vi "ATF-Pumb HW Splitter.vi"(10 "data":T1={"AO config"=[], "AI config"=[], "DI config"=[], "DO config"=[], "TC config"=[], "ACC config"=[], "SG config"=[], "Strain Gauge Settings"={"poisson ratio"=0.3, "nominal gage resistance"=120.0, "gage factor"=2.08}, "Bridge Settings"={"voltage excitation value"=3.3, "voltage excitation source"=10200, "initial bridge voltage"=0.0, "lead wire resistance"=1.7, "strain configuration"=10271}, "Sample Rate"={"AI Sample Rate"=[], "AO Sample Rate"=[], "DI Sample Rate"=[], "TC Sample Rate"=[], "DO Sample Rate"=[], "SG Sample Rate"=[], "ACC Sample Rate"=[]}} {"Bridge Settings"."strain configuration" items=["Full Bridge I"=10183, "Full Bridge II"=10184, "Full Bridge III"=10185, "Half Bridge I"=10188, "Half Bridge II"=10189, "Quarter Bridge I"=10271, "Quarter Bridge II"=10272]; "Bridge Settings"."voltage excitation source" items=["Internal"=10200, "External"=10167, "None"=10230]; "ACC config"."Terminal configuration" items=["default"=-1, "RSE"=10083, "NRSE"=10078, "Differential"=10106, "Pseudodifferential"=12529]; "ACC config"."Sensitivity units" items=["mVolts/g"=12509, "Volts/g"=12510]; "TC config"."type" items=["J"=10072, "K"=10073, "N"=10077, "R"=10082, "S"=10085, "T"=10086, "B"=10047, "E"=10055]; "TC config"."units" items=["Deg C", "Deg F", "Kelvins", "Deg R", "From Custom Scale"]}, 11 "Pumb Expression":string="cRIO") -> (1 "Pumb HW":T1={"AO config"=[], "AI config"=[], "DI config"=[], "DO config"=[], "TC config"=[], "ACC config"=[], "SG config"=[], "Strain Gauge Settings"={"poisson ratio"=0.3, "nominal gage resistance"=120.0, "gage factor"=2.08}, "Bridge Settings"={"voltage excitation value"=3.3, "voltage excitation source"=10200, "initial bridge voltage"=0.0, "lead wire resistance"=1.7, "strain configuration"=10271}, "Sample Rate"={"AI Sample Rate"=[], "AO Sample Rate"=[], "DI Sample Rate"=[], "TC Sample Rate"=[], "DO Sample Rate"=[], "SG Sample Rate"=[], "ACC Sample Rate"=[]}} {"Bridge Settings"."strain configuration" items=["Full Bridge I"=10183, "Full Bridge II"=10184, "Full Bridge III"=10185, "Half Bridge I"=10188, "Half Bridge II"=10189, "Quarter Bridge I"=10271, "Quarter Bridge II"=10272]; "Bridge Settings"."voltage excitation source" items=["Internal"=10200, "External"=10167, "None"=10230]; "ACC config"."Terminal configuration" items=["default"=-1, "RSE"=10083, "NRSE"=10078, "Differential"=10106, "Pseudodifferential"=12529]; "ACC config"."Sensitivity units" items=["mVolts/g"=12509, "Volts/g"=12510]; "TC config"."type" items=["J"=10072, "K"=10073, "N"=10077, "R"=10082, "S"=10085, "T"=10086, "B"=10047, "E"=10055]; "TC config"."units" items=["Deg C", "Deg F", "Kelvins", "Deg R", "From Custom Scale"]}, 3 "Storage HW":T1={"AO config"=[], "AI config"=[], "DI config"=[], "DO config"=[], "TC config"=[], "ACC config"=[], "SG config"=[], "Strain Gauge Settings"={"poisson ratio"=0.3, "nominal gage resistance"=120.0, "gage factor"=2.08}, "Bridge Settings"={"voltage excitation value"=3.3, "voltage excitation source"=10200, "initial bridge voltage"=0.0, "lead wire resistance"=1.7, "strain configuration"=10271}, "Sample Rate"={"AI Sample Rate"=[], "AO Sample Rate"=[], "DI Sample Rate"=[], "TC Sample Rate"=[], "DO Sample Rate"=[], "SG Sample Rate"=[], "ACC Sample Rate"=[]}} {"Bridge Settings"."strain configuration" items=["Full Bridge I"=10183, "Full Bridge II"=10184, "Full Bridge III"=10185, "Half Bridge I"=10188, "Half Bridge II"=10189, "Quarter Bridge I"=10271, "Quarter Bridge II"=10272]; "Bridge Settings"."voltage excitation source" items=["Internal"=10200, "External"=10167, "None"=10230]; "ACC config"."Terminal configuration" items=["default"=-1, "RSE"=10083, "NRSE"=10078, "Differential"=10106, "Pseudodifferential"=12529]; "ACC config"."Sensitivity units" items=["mVolts/g"=12509, "Volts/g"=12510]; "TC config"."type" items=["J"=10072, "K"=10073, "N"=10077, "R"=10082, "S"=10085, "T"=10086, "B"=10047, "E"=10055]; "TC config"."units" items=["Deg C", "Deg F", "Kelvins", "Deg R", "From Custom Scale"]})   [LabVIEW 2022 SP3]
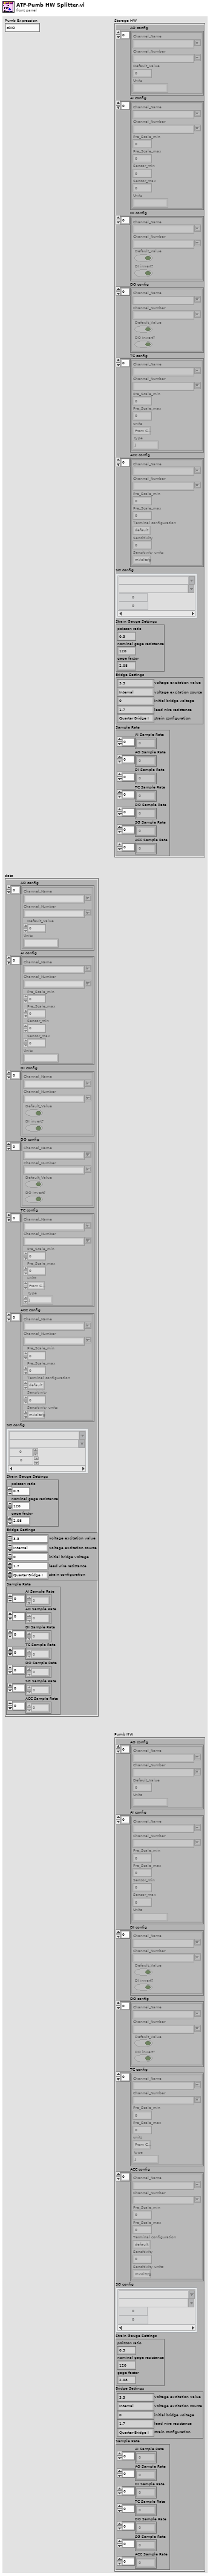
[diagram p1: front panel]
types:
  T1 = cluster{"AO config":cluster{"Channel_Name":string, "Channel_Number":string, "Default_Value":dbl, "Units":string}[], "AI config":cluster{"Channel_Name":string, "Channel_Number":string, "Pre_Scale_min":dbl, "Pre_Scale_max":dbl, "Sensor_min":dbl, "Sensor_max":dbl, "Units":string}[], "DI config":cluster{"Channel_Name":string, "Channel_Number":string, "Default_Value":bool, "DI invert?":bool}[], "DO config":cluster{"Channel_Name":string, "Channel_Number":string, "Default_Value":bool, "DO invert?":bool}[], "TC config":cluster{"Channel_Name":string, "Channel_Number":string, "Pre_Scale_min":dbl, "Pre_Scale_max":dbl, "units":i32, " type":i32}[], "ACC config":cluster{"Channel_Name":string, "Channel_Number":string, "Pre_Scale_min":dbl, "Pre_Scale_max":dbl, "Terminal configuration":i32, "Sensitivity":dbl, "Sensitivity units":i32}[], "SG config":cluster{"Channel_Name":string, "Channel_Number":string, "Pre_Scale_min":dbl, "Pre_Scale_max":dbl}[], "Strain Gauge Settings":cluster{"poisson ratio":dbl, "nominal gage resistance":dbl, "gage factor":dbl}, "Bridge Settings":cluster{"voltage excitation value":dbl, "voltage excitation source":i32, "initial bridge voltage":dbl, "lead wire resistance":dbl, "strain configuration":i32}, "Sample Rate":cluster{"AI Sample Rate":dbl[], "AO Sample Rate":dbl[], "DI Sample Rate":dbl[], "TC Sample Rate":dbl[], "DO Sample Rate":dbl[], "SG Sample Rate":dbl[], "ACC Sample Rate":dbl[]}}
  T2 = cluster{"Channel_Name":string, "Channel_Number":string, "Default_Value":dbl, "Units":string}[]
  T3 = cluster{"Channel_Name":string, "Channel_Number":string, "Pre_Scale_min":dbl, "Pre_Scale_max":dbl, "Sensor_min":dbl, "Sensor_max":dbl, "Units":string}[]
  T4 = cluster{"Channel_Name":string, "Channel_Number":string, "Default_Value":bool, "DI invert?":bool}[]
  T5 = cluster{"Channel_Name":string, "Channel_Number":string, "Default_Value":bool, "DO invert?":bool}[]
  T6 = cluster{"Channel_Name":string, "Channel_Number":string, "Pre_Scale_min":dbl, "Pre_Scale_max":dbl, "units":i32, " type":i32}[]
  T7 = cluster{"Channel_Name":string, "Channel_Number":string, "Pre_Scale_min":dbl, "Pre_Scale_max":dbl, "Terminal configuration":i32, "Sensitivity":dbl, "Sensitivity units":i32}[]
  T8 = cluster{"Channel_Name":string, "Channel_Number":string, "Pre_Scale_min":dbl, "Pre_Scale_max":dbl}[]
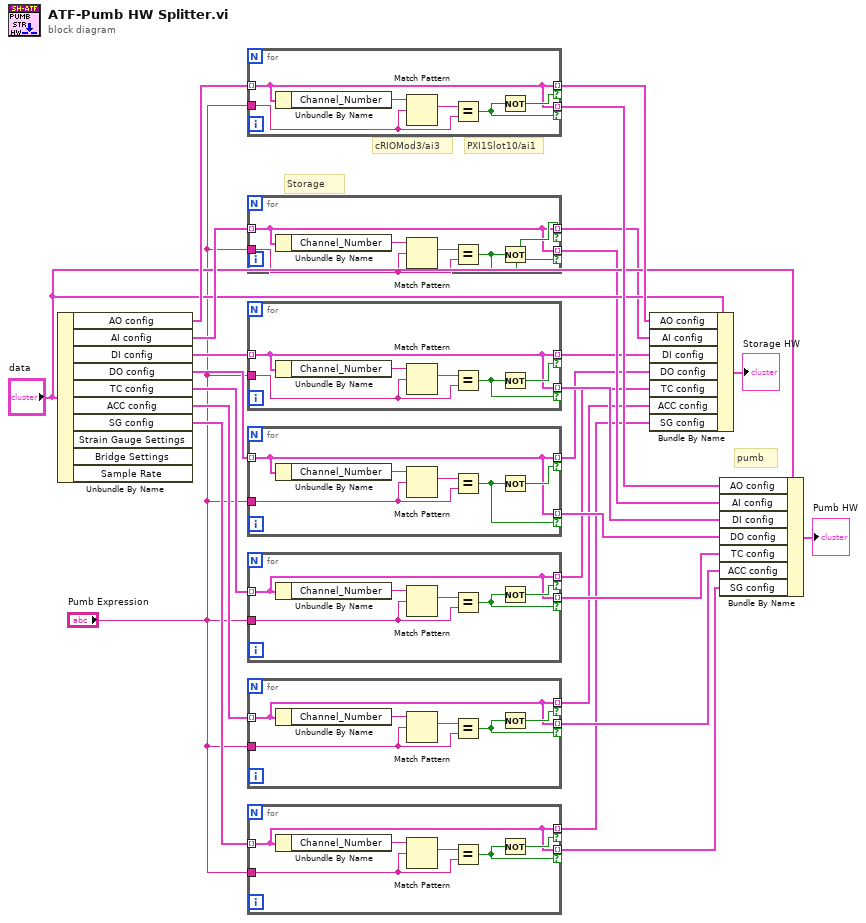
[diagram p0: block diagram]
diagram:
  # "Storage"
  # "pumb"
  # "cRIOMod3/ai3"
  # "PXI1Slot10/ai1"
  n1 = Unbundle By Name("data") -> ("AO config"=w25:T2, "AI config"=w24:T3, "DI config"=w18:T4, "DO config"=w15:T5, "TC config"=w12:T6, "ACC config"=w9:T7, "SG config"=w6:T8)  [unwired: 3 out]
  n2 = for {
    tunnel: w25 -> [w26] mode=indexing
    tunnel: [w26] -> w23 mode=indexing if=w29
    tunnel: [w26] -> w22 mode=indexing if=w28
    tunnel: "Pumb Expression" -> [w27]
    n3 = Unbundle By Name(w26) -> ("Channel_Number"=w30:string)
    n4 = Match Pattern(string=w30, regular expression=w27) -> (match substring=w31:string)  [unwired: 1 in, 3 out]
    n5 = Equal?(x=w31, y=w27) -> (x = y?=w29:bool)
    n6 = Not(x=w29) -> (.not. x?=w28:bool)
  }
  n7 = for {
    tunnel: w24 -> [w32] mode=indexing
    tunnel: [w32] -> w20 mode=indexing if=w35
    tunnel: [w32] -> w19 mode=indexing if=w34
    tunnel: "Pumb Expression" -> [w33]
    n8 = Unbundle By Name(w32) -> ("Channel_Number"=w36:string)
    n9 = Match Pattern(string=w36, regular expression=w33) -> (match substring=w37:string)  [unwired: 1 in, 3 out]
    n10 = Equal?(x=w37, y=w33) -> (x = y?=w35:bool)
    n11 = Not(x=w35) -> (.not. x?=w34:bool)
  }
  n12 = for {
    tunnel: w18 -> [w38] mode=indexing
    tunnel: [w38] -> w17 mode=indexing if=w41
    tunnel: [w38] -> w16 mode=indexing if=w40
    tunnel: "Pumb Expression" -> [w39]
    n13 = Unbundle By Name(w38) -> ("Channel_Number"=w42:string)
    n14 = Match Pattern(string=w42, regular expression=w39) -> (match substring=w43:string)  [unwired: 1 in, 3 out]
    n15 = Equal?(x=w43, y=w39) -> (x = y?=w41:bool)
    n16 = Not(x=w41) -> (.not. x?=w40:bool)
  }
  n17 = for {
    tunnel: w15 -> [w44] mode=indexing
    tunnel: [w44] -> w14 mode=indexing if=w47
    tunnel: [w44] -> w13 mode=indexing if=w46
    tunnel: "Pumb Expression" -> [w45]
    n18 = Unbundle By Name(w44) -> ("Channel_Number"=w48:string)
    n19 = Match Pattern(string=w48, regular expression=w45) -> (match substring=w49:string)  [unwired: 1 in, 3 out]
    n20 = Equal?(x=w49, y=w45) -> (x = y?=w47:bool)
    n21 = Not(x=w47) -> (.not. x?=w46:bool)
  }
  n22 = for {
    tunnel: w12 -> [w50] mode=indexing
    tunnel: [w50] -> w10 mode=indexing if=w53
    tunnel: [w50] -> w11 mode=indexing if=w52
    tunnel: "Pumb Expression" -> [w51]
    n23 = Unbundle By Name(w50) -> ("Channel_Number"=w54:string)
    n24 = Match Pattern(string=w54, regular expression=w51) -> (match substring=w55:string)  [unwired: 1 in, 3 out]
    n25 = Equal?(x=w55, y=w51) -> (x = y?=w53:bool)
    n26 = Not(x=w53) -> (.not. x?=w52:bool)
  }
  n27 = for {
    tunnel: w9 -> [w56] mode=indexing
    tunnel: [w56] -> w8 mode=indexing if=w59
    tunnel: [w56] -> w7 mode=indexing if=w58
    tunnel: "Pumb Expression" -> [w57]
    n28 = Unbundle By Name(w56) -> ("Channel_Number"=w60:string)
    n29 = Match Pattern(string=w60, regular expression=w57) -> (match substring=w61:string)  [unwired: 1 in, 3 out]
    n30 = Equal?(x=w61, y=w57) -> (x = y?=w59:bool)
    n31 = Not(x=w59) -> (.not. x?=w58:bool)
  }
  n32 = for {
    tunnel: w6 -> [w62] mode=indexing
    tunnel: [w62] -> w3 mode=indexing if=w65
    tunnel: [w62] -> w4 mode=indexing if=w64
    tunnel: "Pumb Expression" -> [w63]
    n33 = Unbundle By Name(w62) -> ("Channel_Number"=w66:string)
    n34 = Match Pattern(string=w66, regular expression=w63) -> (match substring=w67:string)  [unwired: 1 in, 3 out]
    n35 = Equal?(x=w67, y=w63) -> (x = y?=w65:bool)
    n36 = Not(x=w65) -> (.not. x?=w64:bool)
  }
  n37 = Bundle By Name(cluster="data", "AO config"=w22, "AI config"=w19, "DI config"=w16, "DO config"=w13, "TC config"=w11, "ACC config"=w7, "SG config"=w4) -> (→"Storage HW":T1)
  n38 = Bundle By Name(cluster="data", "AO config"=w23, "AI config"=w20, "DI config"=w17, "DO config"=w14, "TC config"=w10, "ACC config"=w8, "SG config"=w3) -> (→"Pumb HW":T1)
